vi "GetLength.vi"(8 "error in (no error)":errorcluster, 11 "VISA resource name":refnum<visa-resource-name>="COM3") -> (0 "error out":errorcluster, 2 "SensorLength":dbl)   [LabVIEW 2017]
uses:
  <vilib>/Instr/_visa.llb/VISA Configure Serial Port (Instr).vi
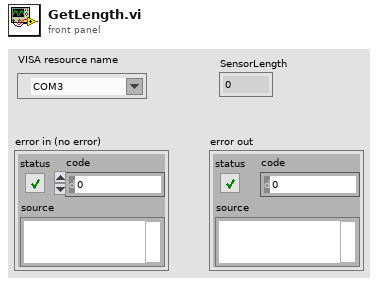
[diagram p1: front panel]
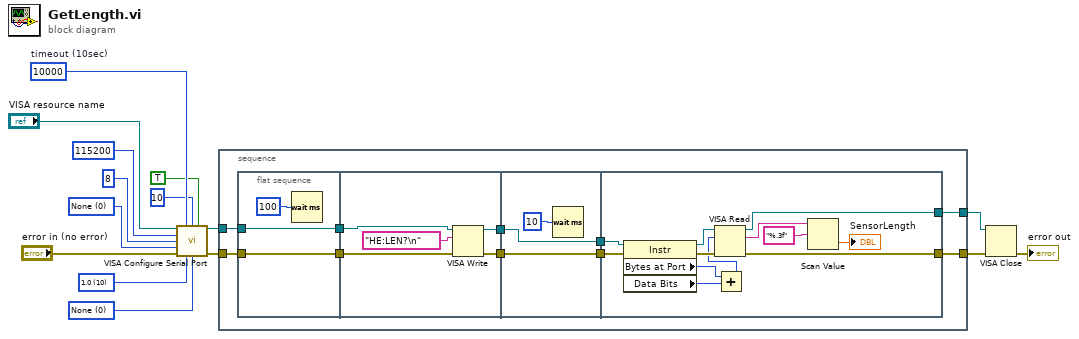
[diagram p0: block diagram]
diagram:
  w5 = u16 0 items=["None"=0, "XON/XOFF"=1, "RTS/CTS"=2, "DTR/DSR"=4] ("flow control")
  w6 = u16 10 items=["1.0"=10, "1.5"=15, "2.0"=20] ("stop bits")
  w8 = u16 0 items=["None", "Odd", "Even", "Mark", "Space"] ("parity")
  w13 = u32 10000  # timeout (10sec)
  n1 = call-poly "VISA Configure Serial Port"("VISA resource name"="VISA resource name", "timeout (10sec)"=w13, "termination char\n(0xA = '\\n' = LF)"=u8 10 ("termination char\n(0xA = '\\n' = LF)"), "Enable Termination\nChar (T)"=TRUE ("Enable Termination Char (T)"), "baud rate (9600)"=u32 115200 ("baud rate"), "data bits (8)"=u16 8 ("data bits"), "parity (0:none)"=w8, "error in (no error)"="error in (no error)", "stop bits (10: 1 bit)"=w6, "flow control (0:none)"=w5) -> ("VISA resource name out"=w4:refnum<visa-resource-name>, "error out"=w3:errorcluster)  [unwired: 4 in]
  n2 = stacked-sequence {
    tunnel: w4 -> [w20]
    tunnel: w3 -> [w18]
    tunnel: [w21] -> w2
    tunnel: [w19] -> w1
    frame #0 {
      n3 = flat-sequence {
        tunnel: w18 -> [w27]
        tunnel: w20 -> [w28]
        tunnel: [w28] -> w17
        tunnel: [w27] -> w16
        tunnel: [w33] -> w25
        tunnel: [w32] -> w24
        tunnel: w17 -> [w30]
        tunnel: w16 -> [w29]
        tunnel: w25 -> [w36]
        tunnel: [w36] -> w23
        tunnel: w24 -> [w35]
        tunnel: [w35] -> w22
        tunnel: w23 -> [w48]
        tunnel: w22 -> [w47]
        tunnel: [w44] -> w21
        tunnel: [w43] -> w19
        frame #0 {
          n4 = Wait (ms)(milliseconds to wait=u32 100) -> ()  [unwired: 1 out]
        }
        frame #1 {
          n5 = VISA Write(VISA resource name=w30, write buffer="HE:LEN?\n" ("string to write 2"), error in (no error)=w29) -> (VISA resource name out=w33:refnum<visa-resource-name>, error out=w32:errorcluster)  [unwired: 1 out]
        }
        frame #2 {
          n6 = Wait (ms)(milliseconds to wait=u32 10) -> ()  [unwired: 1 out]
        }
        frame #3 {
          n7 = property class="Instr"(reference=w48, error in=w47) -> (reference out=w45:refnum<visa-resource-name>, error out=w46:errorcluster, "Bytes at Port"=w39:u32, "Data Bits"=w37:u16)
          n8 = Add(x=w39, y=w37) -> (x+y=w38:u32)
          n9 = VISA Read(VISA resource name=w45, byte count=w38, error in (no error)=w46) -> (VISA resource name out=w43:refnum<visa-resource-name>, read buffer=w42:string, error out=w44:errorcluster)  [unwired: 1 out]
          n10 = Scan Value(string=w42, format string="%.3f") -> (value=→"SensorLength":dbl)  [unwired: 1 in, 1 out]
        }
      }
    }
  }
  n11 = VISA Close(VISA resource name=w1, error in (no error)=w2) -> (error out=→"error out":errorcluster)
